vi "create2.vi"(6 "actual y size":i32, 9 "center":i32, 10 "X size":i32, 11 "max Y size":i32) -> (1 "size":i32, 3 "Array":i32[][](array[numeric]))   [LabVIEW 2011]
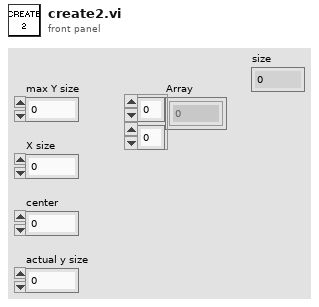
[diagram p1: front panel]
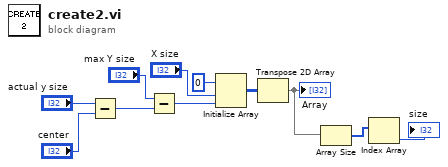
[diagram p0: block diagram]
diagram:
  n1 = Subtract(x="actual y size", y="center") -> (x-y=w6:i32)
  n2 = Subtract(x="max Y size", y=w6) -> (x-y=w4:i32)
  n3 = Initialize Array(0, "X size", w4) -> (w7:i32[][])
  n4 = Transpose 2D Array(2D array=w7) -> (transposed array=w3:i32[][])
  "Array" <- w3
  n5 = Array Size(array=w3) -> (size(s)=w2:i32[])
  n6 = Index Array(array=w2) -> (element=→"size":i32)  [unwired: 1 in]
